vi "ConfChannelMetodo.vi"(7 "Enable Channel (True)":bool=TRUE, 8 "error in (no error)":errorcluster, 10 "ConfigChannel":T1={"Probe Attenuation (10: 10X)"=10, "Vertical Range (10.0 V/div)"=10.0, "Vertical Offset (0.0 divs)"=0.0, "Bandwidth (0: MAX Bandwidth)"=0, "Channel (0: Channel 1)"=0, "Vertical Coupling (1: DC)"=1} {"Vertical Coupling (1: DC)" items=["AC", "DC", "Ground"]; "Channel (0: Channel 1)" items=["Channel 1", "Channel 2", "Channel 3", "Channel 4", "Math", "Reference A", "Reference B", "Reference C", "Reference D"]; "Bandwidth (0: MAX Bandwidth)" items=["MAX Bandwidth", "Unlimited"]; "Probe Attenuation (10: 10X)" items=["1"=1, "10"=10, "20"=20, "50"=50, "100"=100, "500"=500, "1000"=1000]}, 11 "TektroniksTDS in":refnum<class "TektroniksTDS.lvclass">) -> (0 "error out":errorcluster, 3 "TektroniksTDS out":refnum<class "TektroniksTDS.lvclass">)   [LabVIEW 2020, in "TektroniksTDS.lvclass"]
uses:
  TektroniksTDS.lvclass
  TektroniksTDS.lvclass/TektroniksTDS.ctl
  <instrlib>/Tektronix TDS 200 1000 2000 Series/Tektronix TDS 200 1000 2000 Series.lvlib
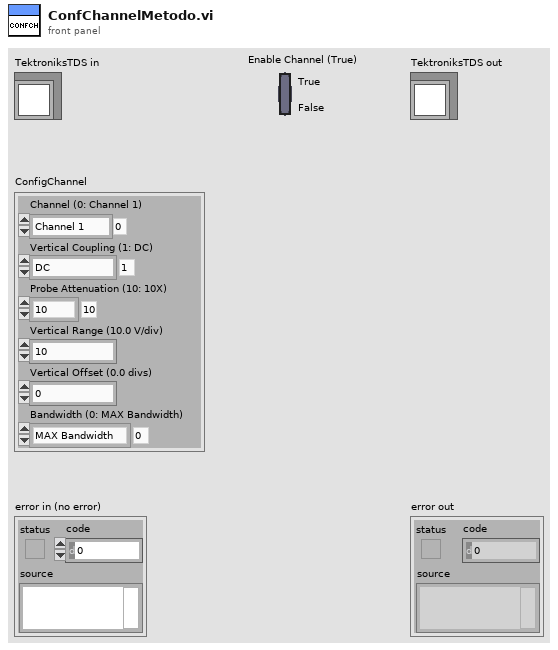
[diagram p1: front panel]
types:
  T1 = cluster{"Probe Attenuation (10: 10X)":i32, "Vertical Range (10.0 V/div)":dbl, "Vertical Offset (0.0 divs)":dbl, "Bandwidth (0: MAX Bandwidth)":i32, "Channel (0: Channel 1)":i32, "Vertical Coupling (1: DC)":i32}
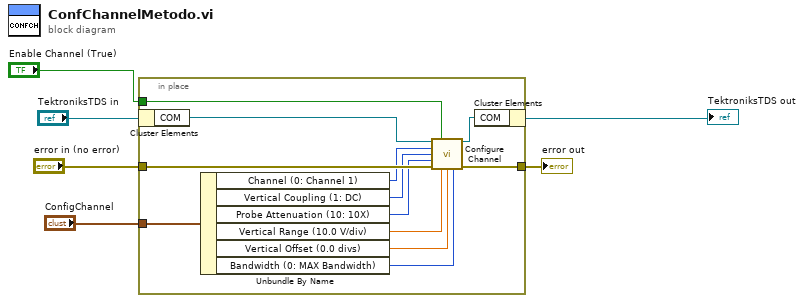
[diagram p0: block diagram]
diagram:
  n1 = in-place {
    in-place-border: "Enable Channel (True)" -> [w18]
    in-place-border: [w15] -> w4
    in-place-border: "error in (no error)" -> [w14]
    in-place-border: "ConfigChannel" -> [w13]
    n2 = in-place-cluster #1("TektroniksTDS in") -> ("COM"=w17:refnum<visa-resource-name>)
    n3 = Unbundle By Name(w13) -> ("Channel (0: Channel 1)"=w12:i32, "Vertical Coupling (1: DC)"=w11:i32, "Probe Attenuation (10: 10X)"=w10:i32, "Vertical Range (10.0 V/div)"=w9:dbl, "Vertical Offset (0.0 divs)"=w8:dbl, "Bandwidth (0: MAX Bandwidth)"=w7:i32)
    n4 = call <instrlib>:"Configure Channel.vi"("VISA resource name"=w17, "Enable Channel (True)"=w18, "Channel (0: Channel 1)"=w12, "Vertical Coupling (1: DC)"=w11, "Probe Attenuation (10: 10X)"=w10, "error in (no error)"=w14, "Vertical Range (10.0 V/div)"=w9, "Vertical Offset (0.0 divs)"=w8, "Bandwidth (0: MAX Bandwidth)"=w7) -> ("VISA resource name out"=w16:refnum<visa-resource-name>, "error out"=w15:errorcluster)  [unwired: 5 in]
    n5 = in-place-cluster #1("COM"=w16) -> (→"TektroniksTDS out":refnum<class "TektroniksTDS.lvclass">)
  }
  "error out" <- w4
